vi "GetGearManipulatorOpenClose.vi"() -> (3 "Gear Manipulator Open Close":enum16{"Open", "Close"}(ring))   [LabVIEW 2016, in "Gear Manipulator.lvclass"]
uses:
  Gear Manipulator.lvclass
  Gear Manipulator.lvclass/Gear Manipulator.ctl
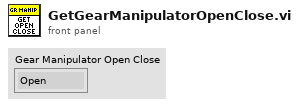
[diagram p1: front panel]
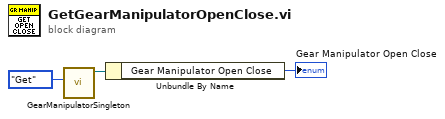
[diagram p0: block diagram]
diagram:
  n1 = call "GearManipulatorSingleton.vi"("Get/Set"=enum16{"Get", "Set"}."Get") -> ("Gear Manipulator.lvclass"=w2:refnum<class "Gear Manipulator.lvclass">)  [unwired: 9 in, 1 out]
  n2 = Unbundle By Name(w2) -> ("Gear Manipulator Open Close"=→"Gear Manipulator Open Close":enum16{"Open", "Close"})
